vi "initialise.vi"(8 "error in (no error)":errorcluster, 11 "GenericPlugin in":refnum<class "FPGAWrapperRK110909Throughput.lvclass">) -> (0 "error out":errorcluster, 3 "GenericPlugin out":refnum<class "FPGAWrapperRK110909Throughput.lvclass">)   [LabVIEW 2010, in "FPGAWrapperRK110909Throughput.lvclass"]
doc: "The dynamic dispatch-version of this VI initalises the plug-in object by allocating and initalising any dynamic resources need."
uses:
  FPGAWrapperRK110909Throughput.lvclass
  GenericFPGAWrapper/GenericFPGAWrapper/GenericFPGAWrapper.lvclass
  <vilib>/userDefined/High Color/nirio_resource_hc.ctl
  FPGA_reference.ctl
  <vilib>/rvi/interface/nirviOpenFPGA/nirviOpenFPGA.xnode
  FPGA Bitfiles/FPGAWrapperRK110_FPGATarget_FPGAThroughput_607C5DD5.lvbitx
  <vilib>/rvi/ClientSDK/nirviWhatTheDeviceIsDoing.ctl
  <vilib>/rvi/interface/nirviMethod/nirviMethod.xnode
  <vilib>/FPGAPlugInAG/PXI-7813R/niLvFpga_Open_PXI-7813R.vi
  <vilib>/rvi/interface/common/dynamic/niFpgaDynamicAddResources.vi
  <vilib>/FPGAPlugInAG/Dynamic/niLvFpga_Reset_Dynamic.vi
  <vilib>/Utility/error.llb/Error Cluster From Error Code.vi
  NiFpgaLv.dll
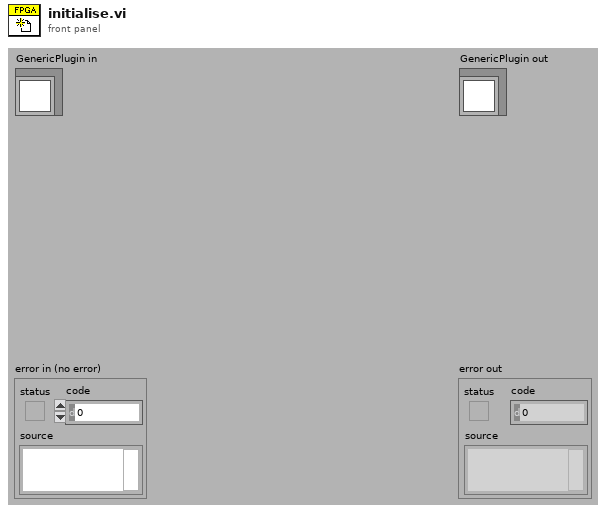
[diagram p1: front panel]
types:
  T1 = typedef "nirio_resource_hc.ctl" = tag
  T2 = typedef "FPGAWrapperRK110909Throughput.lvclass/FPGA_reference.ctl" = refnum<k20>
  T3 = typedef "nirviWhatTheDeviceIsDoing.ctl" = enum32{"nothing", "something other than LabVIEW FPGA", "FPGA interface", "interactive", "emulation"}
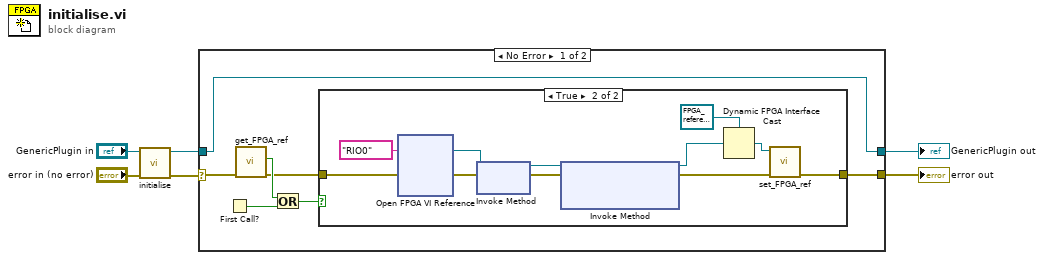
[diagram p0: block diagram]
diagram:
  n1 = call-parent "initialise.vi"("error in (no error)"="error in (no error)", "GenericPlugin in"="GenericPlugin in") -> ("error out"=w4:errorcluster, "GenericPlugin out"=w3:refnum<class "FPGAWrapperRK110909Throughput.lvclass">)  [unwired: 8 in]
  n2 = case shown="No Error" w4 {
    selector: w4 -> [w13 w127]
    tunnel: w3 -> [w7 w126]
    tunnel: [w8 w127] -> w2
    tunnel: [w7 w126] -> w1
    frame No Error {
      n3 = First Call?() -> (First Call?: T/F=w11:bool)
      n4 = call "get_FPGA_ref.vi"("error in"=w13) -> ("error out"=w9:errorcluster, "Is empty?"=w12:bool)  [unwired: 8 in, 1 out]
      n5 = Or(x=w12, y=w11) -> (x .or. y?=w10:bool)
      n6 = case shown="True" w10 {
        tunnel: w9 -> [w14 w25]
        tunnel: [w14 w16] -> w8
        frame False {
        }
        frame True {
          n7 = xnode "Open FPGA VI Reference"("error in"=w25, "resource name"=T1 "RIO0") -> ("FPGA VI Reference Out"=w23:refnum<k20>, "error out"=w24:errorcluster)
          n8 = xnode "Invoke Method"("FPGA VI Reference In"=w23, "error in"=w24) -> ("FPGA VI Reference Out"=w21:refnum<k20>, "error out"=w22:errorcluster)
          n9 = xnode "Invoke Method"("FPGA VI Reference In"=w21, "error in"=w22) -> ("FPGA VI Reference Out"=w20:refnum<k20>, "error out"=w19:errorcluster)  [unwired: 1 in]
          n10 = Dynamic FPGA Interface Cast(Session In=T2 refnum ("FPGA Interface"), Type=w20) -> (Session Out=w17:T2)
          n11 = call "set_FPGA_ref.vi"("error in"=w19, "FPGA Reference"=w17) -> ("error out"=w16:errorcluster)  [unwired: 9 in]
        }
      }
    }
    frame Error {
    }
  }
  "error out" <- w2
  "GenericPlugin out" <- w1
